vi "ch config to senser config.vi"(11 "configtable":T3 {"CHS"."display" format="%b"}) -> (3 "senser out":T1(array[cluster]))   [LabVIEW 2011]
uses:
  singlechtype.ctl
  CHS.ctl
  contable.ctl
panel:
  in  "Sensor":T2={"manner"=enum."线性", "data"=[], "Value max"=0.0, "Value min"=0.0, "sensorID"="", "signal type"="", "unit"=""}
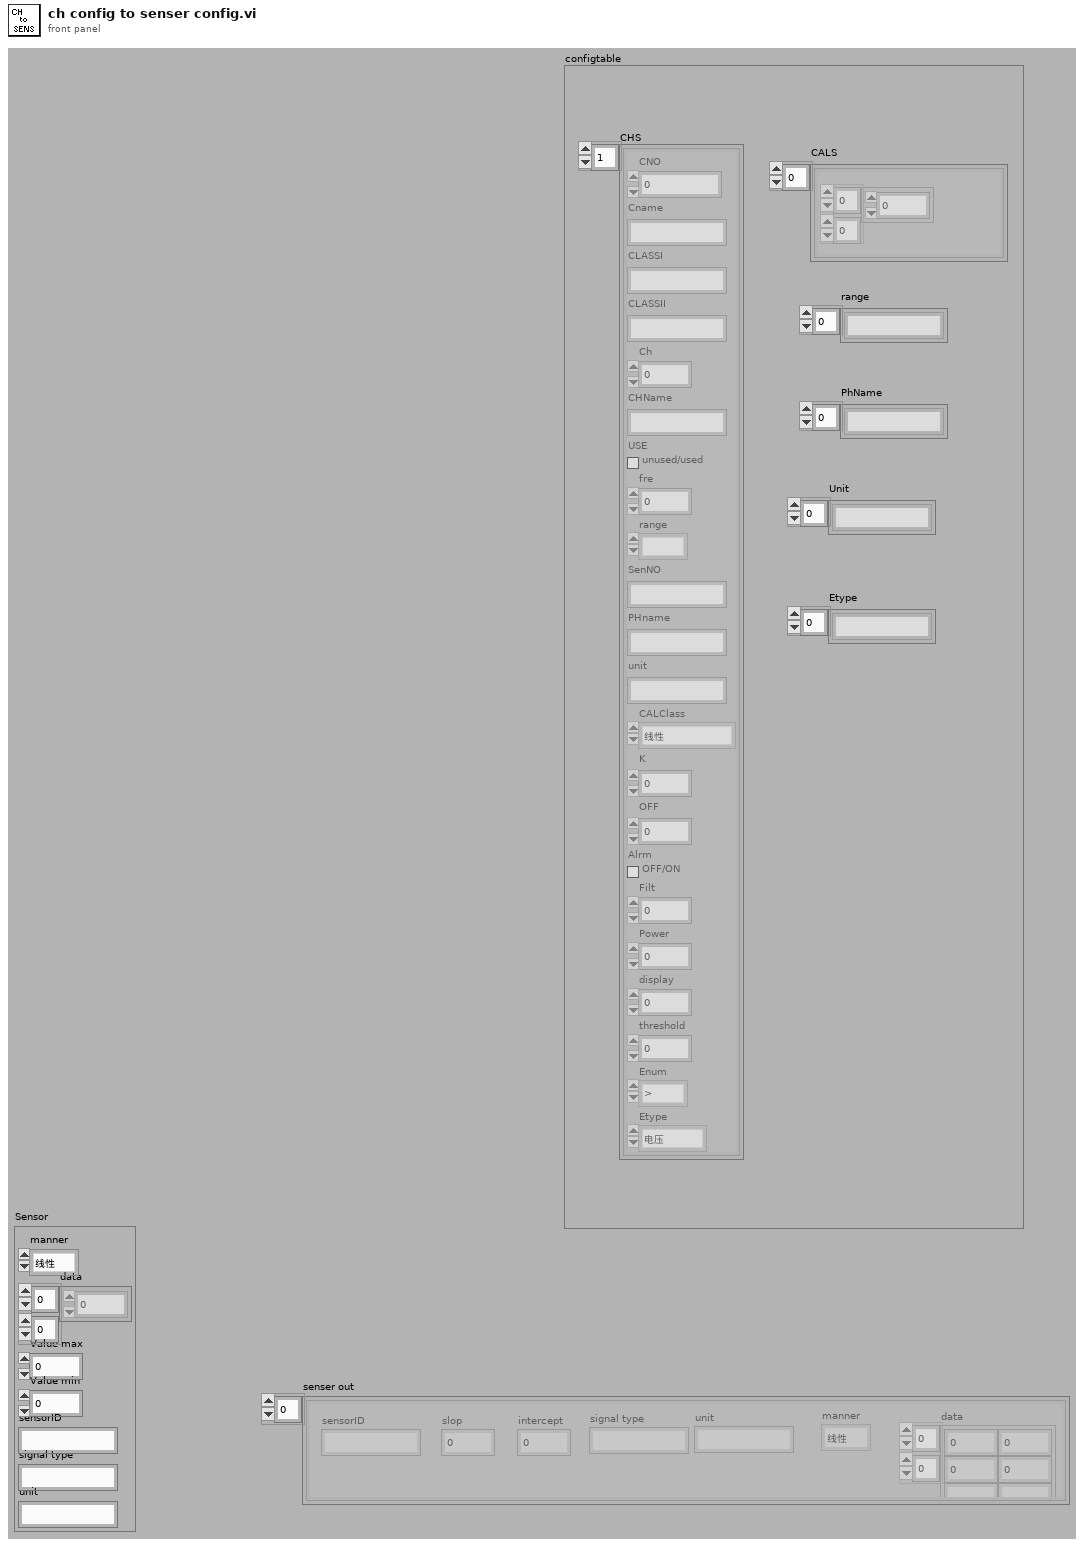
[diagram p1: front panel]
types:
  T1 = cluster{"manner":enum16{"线性", "查表"}, "data":dbl[][], "slop":dbl, "intercept":dbl, "sensorID":string, "signal type":string, "unit":string}[]
  T2 = cluster{"manner":enum16{"线性", "查表"}, "data":dbl[][], "Value max":dbl, "Value min":dbl, "sensorID":string, "signal type":string, "unit":string}
  T3 = typedef "contable.ctl" = cluster{"CHS":T4, "CALS":cluster{"Array":dbl[][]}[], "range":string[], "PhName":string[], "Unit":string[], "Etype":string[]}
  T4 = typedef "CHS.ctl" = T5[]
  T5 = typedef "singlechtype.ctl" = cluster{"CNO":u8, "Cname":string, "CLASSI":string, "CLASSII":string, "Ch":u8, "CHName":string, "USE":bool, "fre":dbl, "range":enum16{""}, "SenNO":string, "PHname":string, "unit":string, "CALClass":enum8{"线性", "查表", "公式"}, "K":dbl, "OFF":dbl, "Alrm":bool, "Filt":dbl, "Power":u8, "display":u8, "threshold ":dbl, "Enum":enum16{">", ">=", "<", "<=", "<>(在范围内）", "><（在范围外）"}, "Etype":enum16{"电压", "电流", "电阻", "热电偶K", "热电偶T"}}
  T6 = cluster{"manner":enum16{"线性", "查表"}, "data":dbl[][], "Value max":dbl, "Value min":dbl, "sensorID":string, "signal type":string, "unit":string}[]
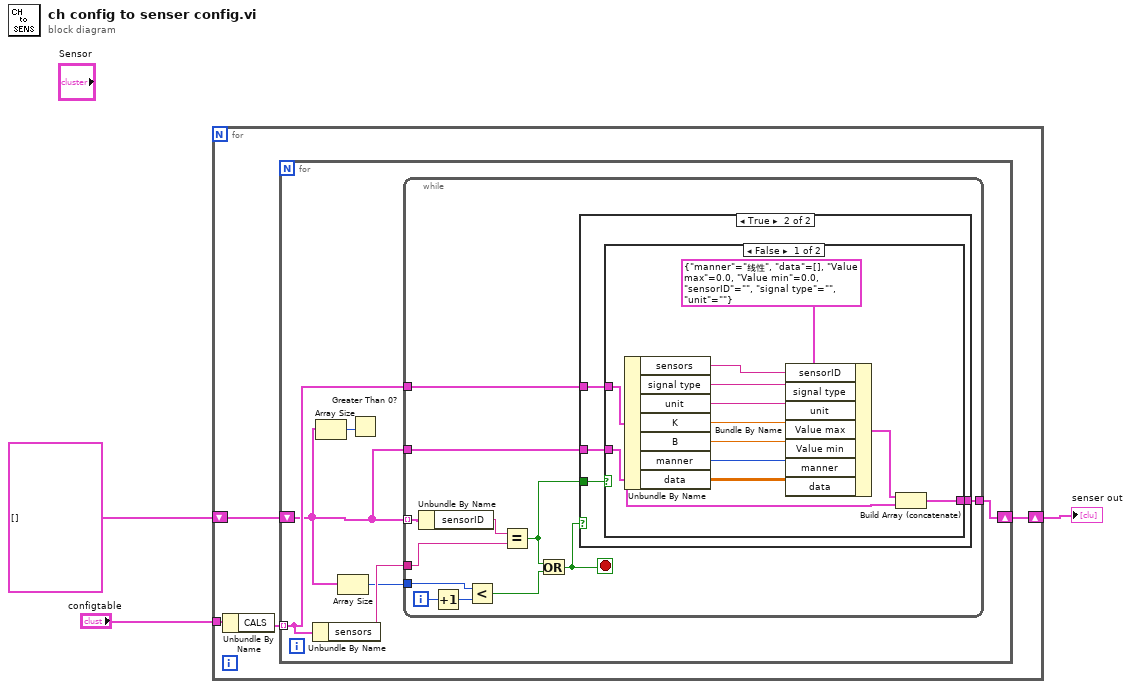
[diagram p0: block diagram]
diagram:
  n1 = for {
    tunnel: "configtable" -> [w7]
    shift-right: [w4] -> w1
    shift-left: T6 [] -> [w5]
    n2 = Unbundle By Name(w7) -> ("CALS"=w6:cluster{"Array":dbl[][]}[])
    n3 = for {
      tunnel: w6 -> [w11] mode=indexing
      shift-right: [w10] -> w4
      shift-left: w5 -> [w9]
      n4 = Unbundle By Name(w11) -> ("sensors"=w13:string)
      n5 = Array Size(array=w9) -> (size(s)=w8:i32)
      n6 = Array Size(array=w9) -> (size(s)=w12:i32)
      n7 = Greater Than 0?(x=w8) -> ()  [unwired: 1 out]
      n8 = while {
        tunnel: w9 -> [w25] mode=indexing
        tunnel: w13 -> [w24]
        tunnel: w12 -> [w23]
        tunnel: w9 -> [w18]
        tunnel: w11 -> [w17]
        tunnel: [w16] -> w10
        i -> [w15]
        stop <- w21 stop-if-true
        n9 = Unbundle By Name(w25) -> ("sensorID"=w20:string)
        n10 = Increment(x=w15) -> (x+1=w14:i32)
        n11 = Less?(x=w23, y=w14) -> (x < y?=w22:bool)
        n12 = Equal?(x=w20, y=w24) -> (x = y?=w19:bool)
        n13 = Or(x=w19, y=w22) -> (x .or. y?=w21:bool)
        n14 = case shown="True" w21 {
          tunnel: w18 -> [w26 w29]
          tunnel: w19 -> [_ w30]
          tunnel: w17 -> [_ w28]
          tunnel: [w26 w27] -> w16
          frame False {
          }
          frame True {
            n15 = case shown="False" w30 {
              tunnel: w29 -> [w33 w43]
              tunnel: w28 -> [w42 _]
              tunnel: [w31 w43] -> w27
              frame False {
                n16 = Unbundle By Name(w42) -> ("sensors"=w40:string, "signal type"=w39:string, "unit"=w38:string, "K"=w37:dbl, "B"=w36:dbl, "manner"=w35:enum16{"线性", "查表"}, "data"=w34:dbl[][])
                n17 = Bundle By Name(cluster=T2 {"manner"=enum."线性", "data"=[], "Value max"=0.0, "Value min"=0.0, "sensorID"="", "signal type"="", "unit"=""} ("Sensor"), "sensorID"=w40, "signal type"=w39, "unit"=w38, "Value max"=w37, "Value min"=w36, "manner"=w35, "data"=w34) -> (w32:T2)
                n18 = Build Array (concatenate)(w32, w33) -> (w31:T6)
              }
              frame True {
              }
            }
          }
        }
      }
    }
  }
  "senser out" <- w1
